vi "Check_Lid_Position.vi"(8 "error in (no error)":errorcluster, 10 "Device Name":string="Dev2", 11 "Device/Ports/Lines":string="Dev1/port1/line0") -> (0 "error out":errorcluster, 2 "data":bool)   [LabVIEW 2015]
uses:
  <vilib>/DAQmx/read.llb/DAQmx Read (Digital Bool 1Line 1Point).vi
  <vilib>/DAQmx/create/channels.llb/DAQmx Create Channel (DI-Digital Input).vi
  <vilib>/DAQmx/miscellaneous.llb/DAQmx Fill In Error Info.vi
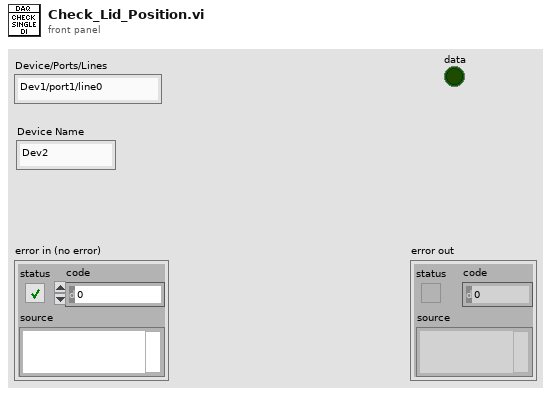
[diagram p1: front panel]
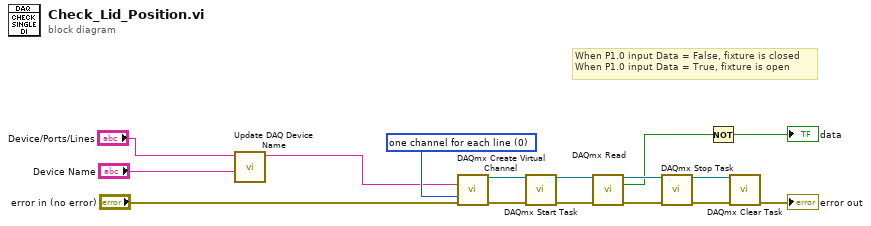
[diagram p0: block diagram]
diagram:
  w16 = 0 items=["one channel for each line", "one channel for all lines"] ("line grouping")
  # "When P1.0 input Data = False, fixture is closed\nWhen P1.0 input Data = True, fixture is open"
  n1 = call "Update DAQ Device Name.vi"("Device Name"="Device Name", "Lines in (String)"="Device/Ports/Lines") -> ("Lines out (DAQmx Physical Channels)"=w2:tag)  [unwired: 9 in]
  n2 = call-poly <vilib>:"DAQmx Create Virtual Channel.vi"("lines"=w2, "line grouping"=w16, "error in"="error in (no error)") -> ("task out"=w15:refnum<k21>, "error out"=w14:errorcluster)  [unwired: 11 in]
  n3 = call <vilib>:"DAQmx Start Task.vi"("task/channels in"=w15, "error in"=w14) -> ("task out"=w13:refnum<k21>, "error out"=w12:errorcluster)  [unwired: 12 in]
  n4 = call-poly <vilib>:"DAQmx Read.vi"("task/channels in"=w13, "error in"=w12) -> ("task out"=w11:refnum<k21>, "data"=w6:bool, "error out"=w10:errorcluster)  [unwired: 11 in]
  n5 = call <vilib>:"DAQmx Stop Task.vi"("task/channels in"=w11, "error in"=w10) -> ("task out"=w9:refnum<k21>, "error out"=w8:errorcluster)  [unwired: 12 in]
  n6 = Not(x=w6) -> (.not. x?=→"data":bool)
  n7 = call <vilib>:"DAQmx Clear Task.vi"("task in"=w9, "error in"=w8) -> ("error out"=→"error out":errorcluster)  [unwired: 13 in]
